vi "test_base64.vi"() -> (3 "All Passed?":bool)   [LabVIEW 2021]
uses:
  src/hashlib.lvlib
panel:
  out "Base64":T1(array[cluster])
  in  "Base64":T2(array[cluster])=[{"Data"="Hello World", "Output"=enum."encode"}, {"Data"="VGhpcyBpcyBhIHRlc3Q=", "Output"=enum."decode"}, {"Data"="\u0000\u0001\u0002\u0003", "Output"=enum."encode"}, {"Data"="The dog jumped over the log", "Output"=enum."encode"}, {"Data"="~!@#$%^&*())_+{}|:\"<>?`1234567890-=[];',./", "Output"=enum."encode"}, {"Data"="1234567890qwertyuiopasdfghjklzxcvbnmQWERTYUIOPASDFGHJKLZXCVBNM", "Output"=enum."encode"}]
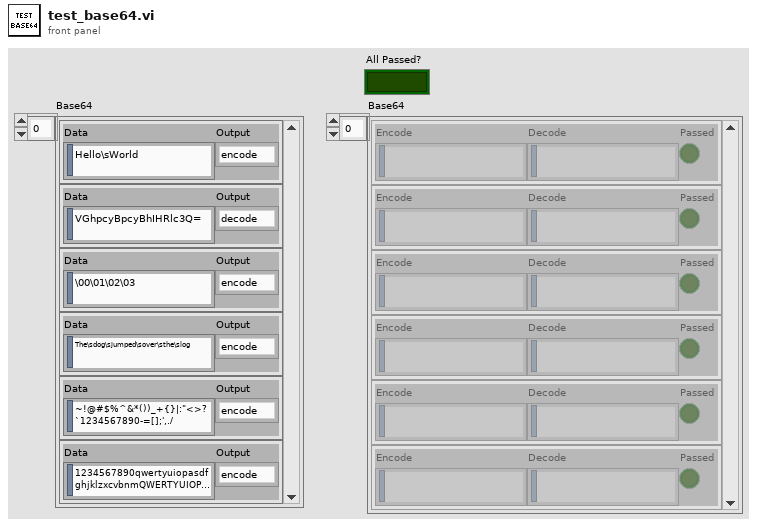
[diagram p1: front panel]
types:
  T1 = cluster{"Encode":string, "Decode":string, "Passed":bool}[]
  T2 = cluster{"Data":string, "Output":enum8{"encode", "decode"}}[]
  T3 = cluster{"Encode":string, "Decode":string, "Passed":bool}
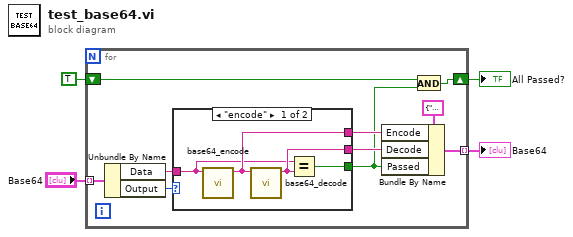
[diagram p0: block diagram]
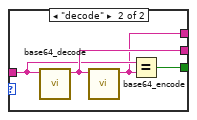
[diagram p2: hidden frame]
diagram:
  n1 = for {
    shift-right: [w13] -> w3
    shift-left: TRUE -> [w14]
    tunnel: "Base64" -> [w12] mode=indexing
    tunnel: [w9] -> w1 mode=indexing
    n2 = Unbundle By Name(w12) -> ("Data"=w11:string, "Output"=w7:enum8{"encode", "decode"})
    n3 = case shown="\"encode\"" w7 {
      tunnel: w11 -> [w16 w20]
      tunnel: [w18 w19] -> w8
      tunnel: [w17 w22] -> w6
      tunnel: [w15 w21] -> w5
      frame "encode" {
        n4 = call "base64_encode.vi"("string"=w16) -> ("base64"=w18:string)  [unwired: 10 in]
        n5 = call "base64_decode.vi"("base64"=w18) -> ("string"=w17:string)  [unwired: 10 in]
        n6 = Equal?(x=w16, y=w17) -> (x = y?=w15:bool)
      }
      frame "decode" {
        n7 = call "base64_decode.vi"("base64"=w20) -> ("string"=w22:string)  [unwired: 10 in]
        n8 = call "base64_encode.vi"("string"=w22) -> ("base64"=w19:string)  [unwired: 10 in]
        n9 = Equal?(x=w20, y=w19) -> (x = y?=w21:bool)
      }
    }
    n10 = Bundle By Name(cluster=T3 {"Encode"="", "Decode"="", "Passed"=FALSE} ("Cluster"), "Encode"=w8, "Decode"=w6, "Passed"=w5) -> (w9:T3)
    n11 = And(x=w14, y=w5) -> (x .and. y?=w13:bool)
  }
  "All Passed?" <- w3
  "Base64" <- w1
